vi "Translate Mirror Data.vi"(11 "Mirror":T2) -> (3 "Mirror String":T1)   [LabVIEW 2016]
uses:
  Mirror Data.ctl
  Messages/Mirror Message Struct.ctl
  Libs/Messages.lvlib
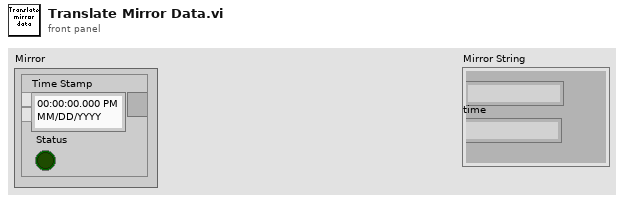
[diagram p1: front panel]
types:
  T1 = typedef "Messages.lvlib/Mirror Message Struct.ctl" = cluster{"status":string, "time":string}
  T2 = typedef "Mirror Data.ctl" = cluster{"Status":bool, "Time Stamp":timestamp}
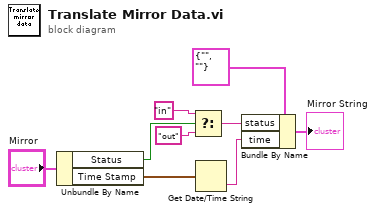
[diagram p0: block diagram]
diagram:
  n1 = Unbundle By Name("Mirror") -> ("Status"=w6:bool, "Time Stamp"=w7:timestamp)
  n2 = Select(t="in", s=w6, f="out") -> (s? t:f=w3:string)
  n3 = Get Date/Time String(seconds (now)=w7) -> (time string=w2:string)  [unwired: 2 in, 1 out]
  n4 = Bundle By Name(cluster=T1 {"status"="", "time"=""} ("ThAr"), "status"=w3, "time"=w2) -> (→"Mirror String":T1)
